vi "QFilter.vi"(8 "error in (no error)":errorcluster, 11 "VISA resource name":refnum<visa-resource-name>) -> (0 "error out":errorcluster, 2 "Filter State":u32(ring) items=["Off", "On"], 3 "VISA resource name out":refnum<visa-resource-name>)   [LabVIEW 2009, in "Newport 1830-C.lvlib"]
doc: "1=use the slow filter to average the last 16 measurements.\n2=use the medium filter to average the last 4 measurements\n3=no averaging is performed"
uses:
  Newport 1830-C.lvlib
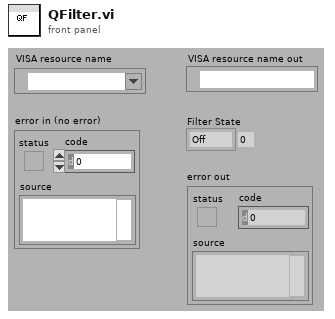
[diagram p1: front panel]
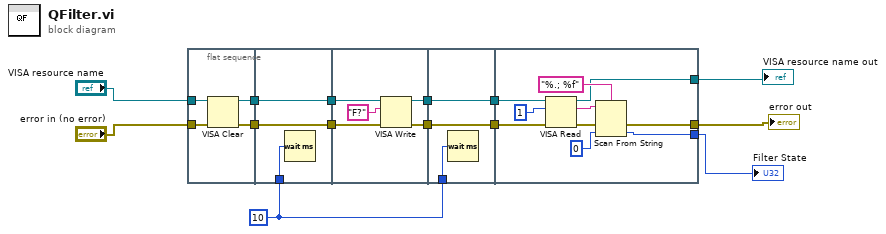
[diagram p0: block diagram]
diagram:
  w6 = u32 10 ("Delay Time (s)")
  n1 = flat-sequence {
    tunnel: [w18] -> w14
    tunnel: [w17] -> w13
    tunnel: "VISA resource name" -> [w16]
    tunnel: "error in (no error)" -> [w15]
    tunnel: [w21] -> w12
    tunnel: w14 -> [w21]
    tunnel: [w20] -> w11
    tunnel: w13 -> [w20]
    tunnel: w6 -> [w19]
    tunnel: [w25] -> w10
    tunnel: [w24] -> w9
    tunnel: w12 -> [w23]
    tunnel: w11 -> [w22]
    tunnel: [w29] -> w8
    tunnel: w10 -> [w29]
    tunnel: w9 -> [w28]
    tunnel: [w28] -> w7
    tunnel: w6 -> [w27]
    tunnel: [w34] -> w4
    tunnel: [w33] -> w3
    tunnel: w8 -> [w32]
    tunnel: w7 -> [w31]
    tunnel: [w30] -> w5
    frame #0 {
      n2 = VISA Clear(VISA resource name=w16, error in (no error)=w15) -> (VISA resource name out=w18:refnum<visa-resource-name>, error out=w17:errorcluster)
    }
    frame #1 {
      n3 = Wait (ms)(milliseconds to wait=w19) -> ()  [unwired: 1 out]
    }
    frame #2 {
      n4 = VISA Write(VISA resource name=w23, write buffer="F?" ("command"), error in (no error)=w22) -> (VISA resource name out=w25:refnum<visa-resource-name>, error out=w24:errorcluster)  [unwired: 1 out]
    }
    frame #3 {
      n5 = Wait (ms)(milliseconds to wait=w27) -> ()  [unwired: 1 out]
    }
    frame #4 {
      n6 = VISA Read(VISA resource name=w32, byte count=u32 1, error in (no error)=w31) -> (VISA resource name out=w34:refnum<visa-resource-name>, read buffer=w36:string, error out=w38:errorcluster)  [unwired: 1 out]
      n7 = Scan From String(format string="%.; %f", input string=w36, error in=w38, default 1=u32 0 ("default value 1")) -> (error out=w33:errorcluster, output 1=w30:u32)  [unwired: 1 in, 2 out]
    }
  }
  "VISA resource name out" <- w4
  "error out" <- w3
  "Filter State" <- w5
